vi "LogStart.vi"(8 "Error In":errorcluster, 10 "Start Time":timestamp, 11 "Base Log Path":path) -> (0 "Error Out":errorcluster, 3 "Log Out":refnum<file>)   [LabVIEW 2012]
uses:
  libs/LV-Utilities/LV-Utilities.lvlib
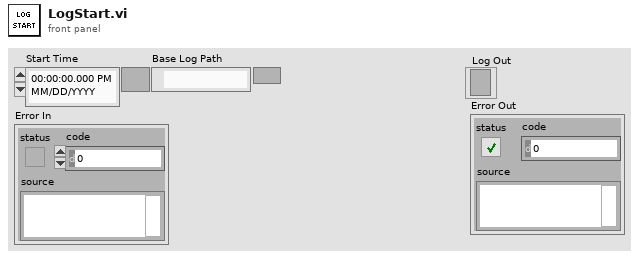
[diagram p1: front panel]
types:
  T1 = enum16{"open", "replace", "create", "open or create", "replace or create", "replace or create with confirmation"}
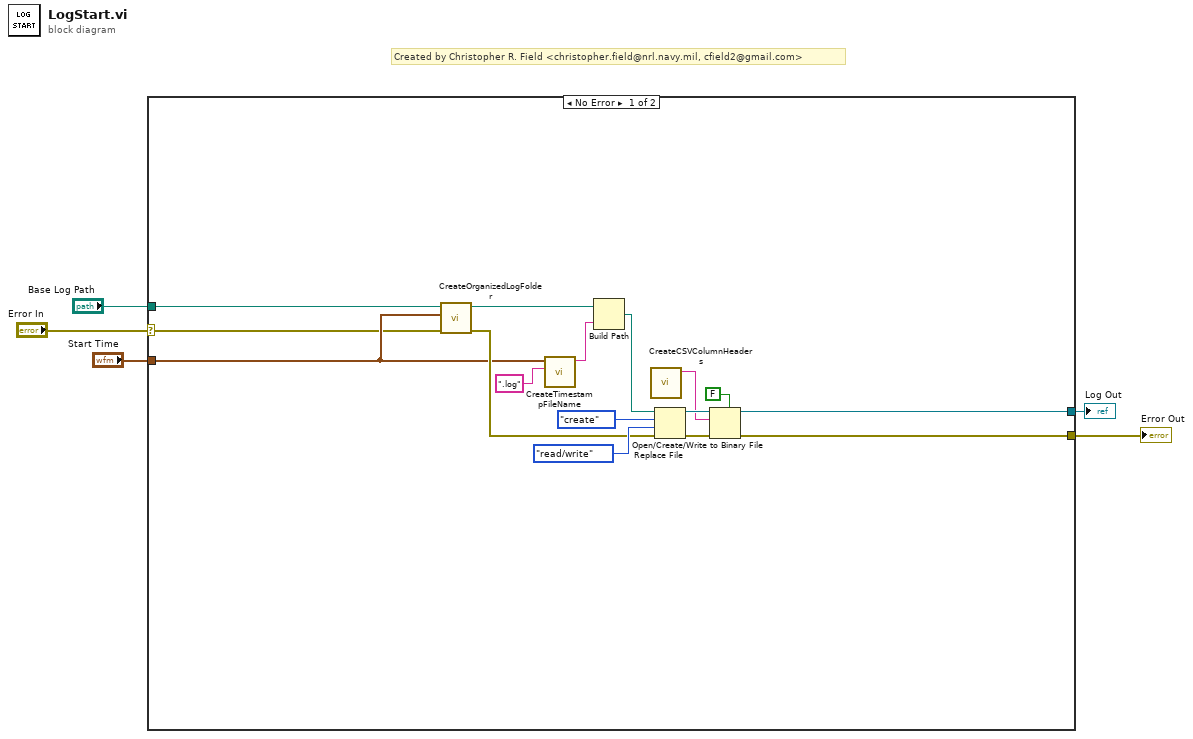
[diagram p0: block diagram]
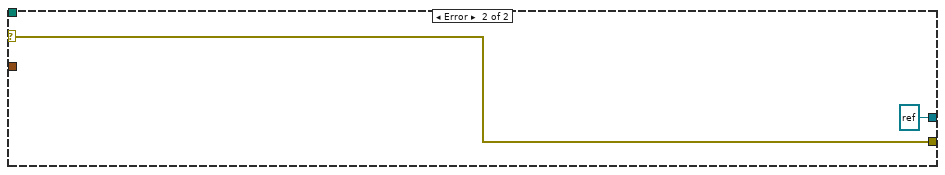
[diagram p2: hidden frame]
diagram:
  # "Created by Christopher R. Field <christopher.field@nrl.navy.mil, cfield2@gmail.com>"
  n1 = case shown="No Error" "Error In" {
    selector: "Error In" -> [w9 w23]
    tunnel: "Start Time" -> [w10 _]
    tunnel: "Base Log Path" -> [w8 _]
    tunnel: [w7 refnum<file> refnum ("refnum out")] -> w2
    tunnel: [w6 w23] -> w1
    frame No Error {
      n2 = call "CreateOrganizedLogFolder.vi"("Error In"=w9, "Time Stamp"=w10, "Base Log Path"=w8) -> ("Error Out"=w11:errorcluster, "Organized Log Path"=w21:path)  [unwired: 7 in]
      n3 = call "CreateTimestampFileName.vi"("File Extension (.csv)"=".log", "Time Stamp"=w10) -> ("Timestamp File Name"=w20:string)  [unwired: 9 in]
      n4 = Build Path(base path=w21, name or relative path=w20) -> (appended path=w16:path)
      n5 = call "CreateCSVColumnHeaders.vi"() -> ("Column Headers"=w12:string)  [unwired: 11 in]
      n6 = Open/Create/Replace File(file path (use dialog)=w16, error in=w11, operation (0:open)=T1."create", access (0:read/write)=enum16{"read/write", "read-only", "write-only"}."read/write") -> (refnum out=w15:refnum<file>, error out=w14:errorcluster)  [unwired: 2 in, 1 out]
      n7 = Write to Binary File(file (use dialog)=w15, data=w12, error in=w14, 5:FALSE ("prepend array or string size? (T)")) -> (refnum out=w7:refnum<file>, error out=w6:errorcluster)  [unwired: 2 in, 1 out]
    }
    frame Error {
    }
  }
  "Log Out" <- w2
  "Error Out" <- w1
